vi "Arm - Joystick Set Output.vi"(8 "error in (no error)":errorcluster, 11 "Buttons":bool[](array[boolean])) -> (0 "error out":errorcluster, 3 "Motor Output":dbl)   [LabVIEW 2014]
uses:
  ArmControlState.ctl
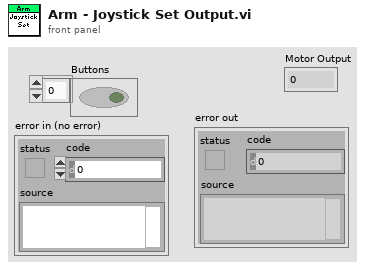
[diagram p1: front panel]
types:
  T1 = typedef "ArmControlState.ctl" = enum16{"Off", "Hold", "Down", "Up"}
  T2 = typedef "WPI_MotorControlDeviceRef.ctl" = cluster{"DeviceStatus":errorcluster, "Type":T3, "PWM":cluster{"Controller":T4, "PWM Channel":T5, "DeadBand":T6}, "CAN":cluster{"Device Number":u8, "Control Mode":T7, "Semaphore":T8, "Max Vout":dbl, "TalonSRX Control Mode":T9}, "Invert":bool, "TransformRef":T10, "InvTransformRef":T10}
  T3 = typedef "WPI_MotorControlType.ctl" = enum16{"PWM", "CAN", "CANTalonSRX"}
  T4 = typedef "FPGA_TypedefDigitalModule.ctl" = enum16{"Controller 1"}
  T5 = typedef "FPGA_DIOPWMChannel.ctl" = enum8{"PWM 0", "PWM 1", "PWM 2", "PWM 3", "PWM 4", "PWM 5", "PWM 6", "PWM 7", "PWM 8", "PWM 9", "PWM MXP 0", "PWM MXP 1", "PWM MXP 2", "PWM MXP 3", "PWM MXP 4", "PWM MXP 5", "PWM MXP 6", "PWM MXP 7", "PWM MXP 8", "PWM MXP 9", "Invalid"}
  T6 = typedef "WPI_PWMDeadband.ctl" = cluster{"Name":string, "maxPositivePwm":i32, "minPositivePwm":i32, "centerPwm":i32, "maxNegativePwm":i32, "minNegativePwm":i32, "angularRange":u16}
  T7 = typedef "WPI_CANJaguar_ControlMode.ctl" = enum8{"Percent VBus", "Current", "Speed", "Position", "Voltage"}
  T8 = typedef "Semaphore RefNum" = refnum<k1>
  T9 = typedef "WPI_CANTalonSRX_APIControlMode.ctl" = enum8{"Percent VBus", "Speed", "Position", "Slave", "Unchanged / Invalid"}
  T10 = typedef "WPI_PWMTransform_ConPane.ctl" = refnum<vi>
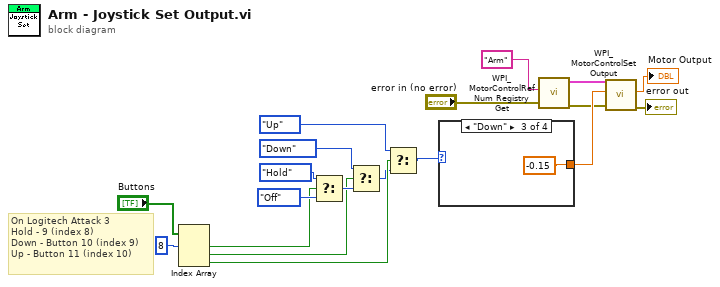
[diagram p0: block diagram]
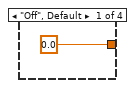
[diagram p2: hidden frame]
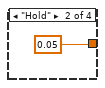
[diagram p3: hidden frame]
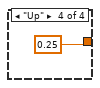
[diagram p4: hidden frame]
diagram:
  # "On Logitech Attack 3\nHold - 9 (index 8)\nDown - Button 10 (index 9)\nUp - Button 11 (index 10)"
  n1 = Index Array(array="Buttons", index #1=8 ("index")) -> (element #1=w9:bool, element #2=w10:bool, element #3=w13:bool)  [unwired: 2 in]
  n2 = Select(t=ArmControlState."Hold", s=w9, f=ArmControlState."Off") -> (s? t:f=w11:T1)
  n3 = Select(t=ArmControlState."Down", s=w10, f=w11) -> (s? t:f=w12:T1)
  n4 = Select(t=ArmControlState."Up", s=w13, f=w12) -> (s? t:f=w18:T1)
  n5 = case shown="\"Down\"" w18 {
    tunnel: [0.0 0.05 -0.15 0.25] -> w19
    frame "Off", Default {
    }
    frame "Hold" {
    }
    frame "Down" {
    }
    frame "Up" {
    }
  }
  n6 = call <vilib>:"WPI_MotorControlRefNum Registry Get.vi"("error in (no error)"="error in (no error)", "refnum name"="Arm") -> ("error out"=w5:errorcluster, "MotorControlDevRef"=w6:T2)  [unwired: 8 in]
  n7 = call <vilib>:"WPI_MotorControlSetOutput.vi"("error in (no error)"=w5, "Output"=w19, "MotorControlDevRef"=w6) -> ("error out"=→"error out":errorcluster, "Motor Output"=→"Motor Output":dbl)  [unwired: 6 in, 1 out]
